vi "Reply.vi"(7 "Sender":refnum<class "Sender.lvclass">, 9 "Is Priority":bool, 10 "Msg":refnum<class "Msg.lvclass">, 11 "Base Actor in":refnum<class "Base Actor.lvclass">) -> (0 "Error out":errorcluster)   [LabVIEW 2020, in "jettl.lvlib" / "Actor.lvlib" / "Base Actor.lvclass"]
uses:
  Base Actor.lvclass
  Sender/Sender/Sender.lvclass
  Msg/Msg.lvclass
  Attributes/Attributes/Attributes.lvclass
  Error/Error.lvlib
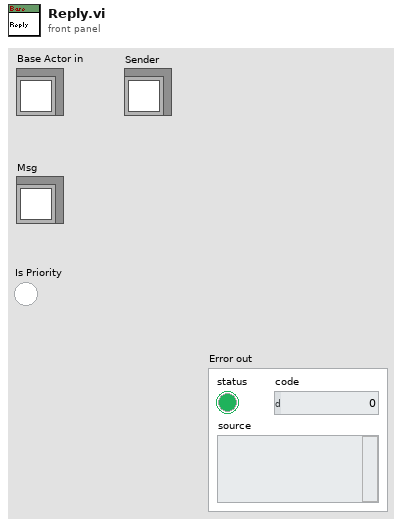
[diagram p1: front panel]
types:
  T1 = typedef "jettl.lvlib/Actor.lvlib/Relation.ctl" = enum16{"Self", "Creator", "Created"}
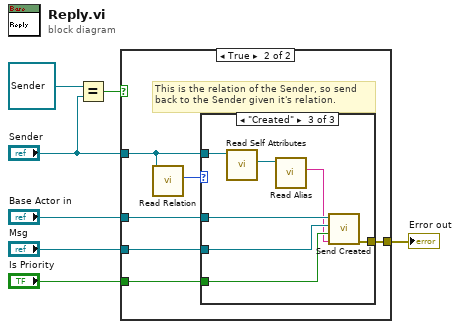
[diagram p0: block diagram]
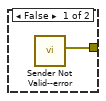
[diagram p2: hidden frame]
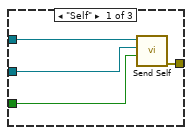
[diagram p3: hidden frame]
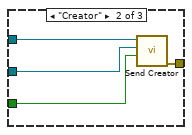
[diagram p4: hidden frame]
diagram:
  n1 = Equal?(x=refnum<class "Sender.lvclass"> refnum ("Sender"), y="Sender") -> (x = y?=w1:bool)
  n2 = case shown="True" w1 {
    tunnel: "Base Actor in" -> [_ w14]
    tunnel: "Msg" -> [_ w13]
    tunnel: "Is Priority" -> [_ w12]
    tunnel: "Sender" -> [_ w11]
    tunnel: [w8 w9] -> w4
    frame False {
      n3 = call "Sender Not Valid--error.vi"() -> ("Error"=w8:errorcluster)  [unwired: 11 in]
    }
    frame True {
      # "This is the relation of the Sender, so send back to the Sender given it's relation."
      n4 = call-dynamic "Read Relation.vi"("Sender in"=w11) -> ("Relation"=w10:T1)  [unwired: 10 in]
      n5 = case shown="\"Created\"" w10 {
        tunnel: w14 -> [w18 w22 w29]
        tunnel: w13 -> [w17 w21 w28]
        tunnel: w12 -> [w16 w20 w27]
        tunnel: w11 -> [_ _ w26]
        tunnel: [w15 w19 w23] -> w9
        frame "Self" {
          n6 = call-dynamic "Send Self.vi"("Is Priority"=w16, "Msg"=w17, "Base Actor in"=w18) -> ("Error out"=w15:errorcluster)  [unwired: 8 in]
        }
        frame "Creator" {
          n7 = call-dynamic "Send Creator.vi"("Is Priority"=w20, "Msg"=w21, "Base Actor in"=w22) -> ("Error out"=w19:errorcluster)  [unwired: 8 in]
        }
        frame "Created" {
          n8 = call-dynamic "Read Self Attributes.vi"("Sender in"=w26) -> ("Self Attributes"=w25:refnum<class "Attributes.lvclass">)  [unwired: 10 in]
          n9 = call-dynamic "Read Alias.vi"("Attributes in"=w25) -> ("Alias"=w24:string)  [unwired: 10 in]
          n10 = call-dynamic "Send Created.vi"("Alias"=w24, "Is Priority"=w27, "Msg"=w28, "Base Actor in"=w29) -> ("Error out"=w23:errorcluster)  [unwired: 7 in]
        }
      }
    }
  }
  "Error out" <- w4
